vi "Drive Axis Modifications.vi"(1 "Drive Info In":T1) -> (0 "Drive Info Out":T1)   [LabVIEW 2013]
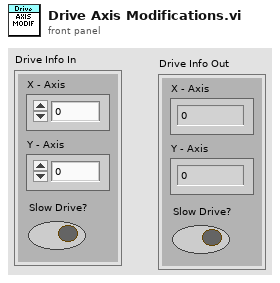
[diagram p1: front panel]
types:
  T1 = cluster{"X - Axis":dbl, "Y - Axis":dbl, "Slow Drive?":bool}
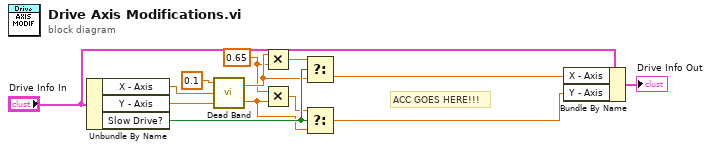
[diagram p0: block diagram]
diagram:
  w3 = 0.65
  # "ACC GOES HERE!!!"
  n1 = Unbundle By Name("Drive Info In") -> ("X - Axis"=w13:dbl, "Y - Axis"=w12:dbl, "Slow Drive?"=w9:bool)
  n2 = call "Dead Band.vi"("Axis 2 In"=w12, "Axis 1 In"=w13, "Dead Band"=0.1) -> ("Axis 2 Out"=w6:dbl, "Axis 1 Out"=w4:dbl)
  n3 = Multiply(x=w4, y=w3) -> (x*y=w5:dbl)
  n4 = Multiply(x=w3, y=w6) -> (x*y=w2:dbl)
  n5 = Select(t=w5, s=w9, f=w4) -> (s? t:f=w8:dbl)
  n6 = Select(t=w2, s=w9, f=w6) -> (s? t:f=w7:dbl)
  n7 = Bundle By Name(cluster="Drive Info In", "X - Axis"=w8, "Y - Axis"=w7) -> (→"Drive Info Out":T1)
